vi "Memory.Pointer.Move Block.vi"   [LabVIEW 2016, in "LabVIEW Memory Manager.lvlib" / "Memory.Pointer.lvclass"]
uses:
  Memory.Pointer.lvclass
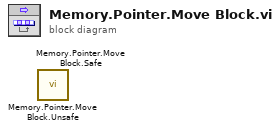
[diagram p0: block diagram]
diagram:
  n1 = call "Memory.Pointer.Move Block.Unsafe.vi"() -> ()  [unwired: 13 in, 3 out]
  n2 = call "Memory.Pointer.Move Block.Safe.vi"() -> ()  [unwired: 13 in, 3 out]
